vi "Initialize Experiment.vi"(7 "lockin address":string, 8 "error in (no error)":errorcluster, 11 "Experiment Comments":string) -> (0 "error out":errorcluster, 1 "Comments":string, 2 "device":string, 3 "path":path)   [LabVIEW 2016, in "Control Experiment.lvclass"]
uses:
  Control Experiment.lvclass
  <userlib>/LevyLab/Lockin-Multichannel/Typedefs/AO-cluster.ctl
  <userlib>/LevyLab/Lockin-Multichannel/Typedefs/AO_Amp-array.ctl
  <userlib>/LevyLab/Lockin-Multichannel/Typedefs/AO_DC-array.ctl
  <userlib>/LevyLab/Lockin-Multichannel/Typedefs/AO_f-array.ctl
  <userlib>/LevyLab/Lockin-Multichannel/Typedefs/AO_phi-array.ctl
  <userlib>/LevyLab/Lockin-Multichannel/Typedefs/Function-array.ctl
  <userlib>/LevyLab/Lockin-Multichannel/Typedefs/Function-enum.ctl
  <userlib>/LevyLab/Lockin-Multichannel/Typedefs/REF-cluster.ctl
  <userlib>/LevyLab/Lockin-Multichannel/Typedefs/REF_f-array.ctl
  <userlib>/LevyLab/Lockin-Multichannel/Typedefs/REF_phi-array.ctl
  <userlib>/LevyLab/Lockin-Multichannel/Typedefs/Sampling.ctl
  <userlib>/LevyLab/Lockin-Multichannel/Typedefs/REF filter-cluster.ctl
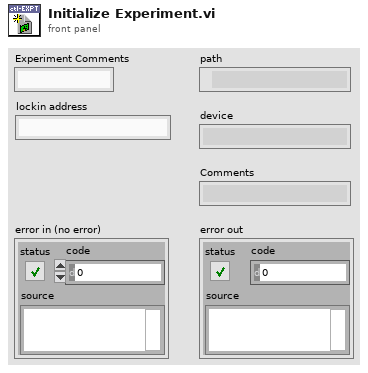
[diagram p1: front panel]
types:
  T1 = typedef "AO-cluster.ctl" = cluster{"AO amp (V)":T2, "AO DC (V)":T3, "AO f (Hz)":T4, "AO phi (°)":T5, "function":T6, "I+":bool[]}
  T2 = typedef "AO_Amp-array.ctl" = dbl[]
  T3 = typedef "AO_DC-array.ctl" = dbl[]
  T4 = typedef "AO_f-array.ctl" = dbl[]
  T5 = typedef "AO_phi-array.ctl" = dbl[]
  T6 = typedef "Function-array.ctl" = T7[]
  T7 = typedef "Function-enum.ctl" = enum16{"Sine", "Triangle", "Square", "Sawtooth"}
  T8 = typedef "REF-cluster.ctl" = cluster{"REF f (Hz)":T9, "REF phi (°)":T10}
  T9 = typedef "REF_f-array.ctl" = dbl[]
  T10 = typedef "REF_phi-array.ctl" = dbl[]
  T11 = typedef "Sampling.ctl" = cluster{"Fs":i32, "#s":i32}
  T12 = typedef "REF filter-cluster.ctl" = cluster{"TC (s)":dbl, "order":i32}
  T13 = cluster{"Channels: AO":T1, "REF config":T8, "sampling":T11, "REF filter":T12}
  T14 = typedef "Control Experiment.lvclass/Control Experiment FGV-cluster.ctl" = cluster{"path":path, "device":string, "user":string, "comments":string, "Lockin Ch":enum16{"1", "2", "3", "4", "5", "6", "7", "8"}[], "Electrode":u32[], "Label":string[], "KH Ch":enum32{"1", "2", "3", "4", "5", "6", "7", "8"}[], "KH Configuration":T15[], "Gain":u32[], "Shunt Resistor":u32[]}
  T15 = typedef "KH7008.lvclass/Input Configuration-Enum.ctl" = enum16{"Ground", "SE+ (-gnd)", "SE- (+gnd)", "Differential"}
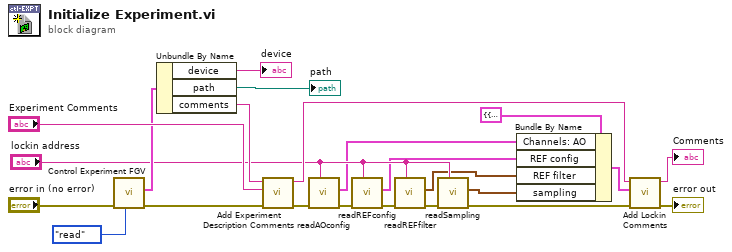
[diagram p0: block diagram]
diagram:
  n1 = call "Control Experiment FGV.vi"("Function"=enum16{"read", "write"}."read", "error in (no error)"="error in (no error)") -> ("error out"=w10:errorcluster, "Cluster out"=w13:T14)  [unwired: 8 in]
  n2 = Unbundle By Name(w13) -> ("device"=→"device":string, "path"=→"path":path, "comments"=w11:string)
  n3 = call "Add Experiment Description Comments.vi"("error in (no error)"=w10, "Experiment Description"="Experiment Comments", "Comments in"=w11) -> ("error out"=w9:errorcluster, "Comments"=w8:string)  [unwired: 6 in]
  n4 = call <userlib>:"readAOconfig.vi"("address"="lockin address", "error in (no error)"=w9) -> ("error out"=w18:errorcluster, "AOconfig"=w1:T1)  [unwired: 8 in]
  n5 = call <userlib>:"readREFconfig.vi"("address"="lockin address", "error in (no error)"=w18) -> ("error out"=w19:errorcluster, "REFconfig"=w2:T8)  [unwired: 8 in]
  n6 = call <userlib>:"readREFfilter.vi"("address"="lockin address", "error in (no error)"=w19) -> ("error out"=w20:errorcluster, "REF filter"=w3:T12)  [unwired: 8 in]
  n7 = call <userlib>:"readSampling.vi"("address"="lockin address", "error in (no error)"=w20) -> ("error out"=w21:errorcluster, "sampling"=w4:T11)  [unwired: 8 in]
  n8 = Bundle By Name(cluster=T13 {"Channels: AO"={"AO amp (V)"=[0.01, 0.0, 0.0, 0.0, 0.0, 0.0, 0.0, 0.0], "AO DC (V)"=[0.0, 0.0, 0.0, 0.0, 0.0, 0.0, 0.0, 0.0], "AO f (Hz)"=[13.1, 13.0, 13.0, 13.0, 13.0, 13.0, 13.0, 13.0], "AO phi (°)"=[0.0, 0.0, 0.0, 0.0, 0.0, 0.0, 0.0, 0.0], "function"=[enum."Sine", enum."Sine", enum."Sine", enum."Sine", enum."Sine", enum."Sine", enum."Sine", enum."Sine"], "I+"=[]}, "REF config"={"REF f (Hz)"=[13.0, 26.0], "REF phi (°)"=[0.0, 0.0, 0.0, 0.0, 0.0, 0.0, 0.0, 0.0]}, "sampling"={"Fs"=204789, "#s"=15753}, "REF filter"={"TC (s)"=0.3, "order"=2}} ("Lockin Configuration"), "Channels: AO"=w1, "REF config"=w2, "REF filter"=w3, "sampling"=w4) -> (w23:T13)
  n9 = call "Add Lockin Comments.vi"("error in (no error)"=w21, "Lockin Configuration"=w23, "Comments in"=w8) -> ("error out"=→"error out":errorcluster, "Comments"=→"Comments":string)  [unwired: 6 in]
